vi "write_filter_spec.vi"(9 "IIR Filter Cluster":T1 {"Forward Coefficients" format="%#_4g"; "Reverse Coefficients" format="%#_4g"}, 11 "File path":path) -> (1 "Output matrix":dbl[][](array[numeric]) format="%0.3f")   [LabVIEW 2010]
uses:
  <vilib>/Utility/file.llb/Write To Spreadsheet File (DBL).vi
panel:
  # "Write out an IIR second order sections filter in the Matlab zpk2sos format.\n\nNote that in Labview terminology, with the transfer function b/a, b (the numerator) is  the \"Forward Coefficients\" and a (the denominator) is the \"Reverse Coefficients\"."
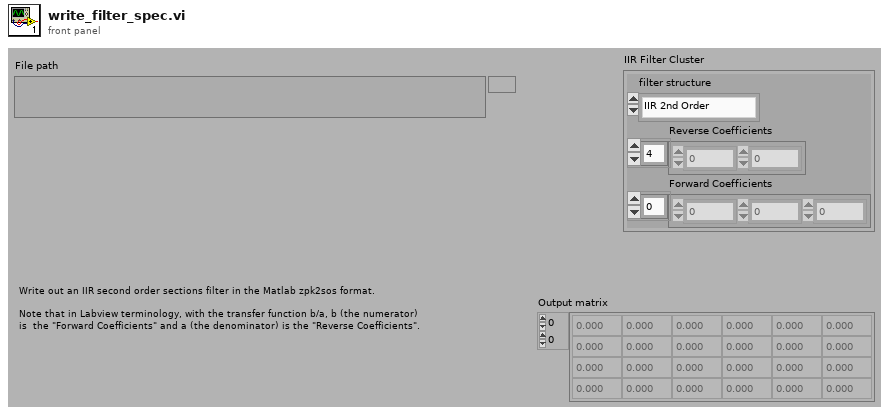
[diagram p1: front panel]
types:
  T1 = cluster{"filter structure":enum32{"IIR 2nd Order", "IIR 4th Order"}, "Reverse Coefficients":dbl[], "Forward Coefficients":dbl[]}
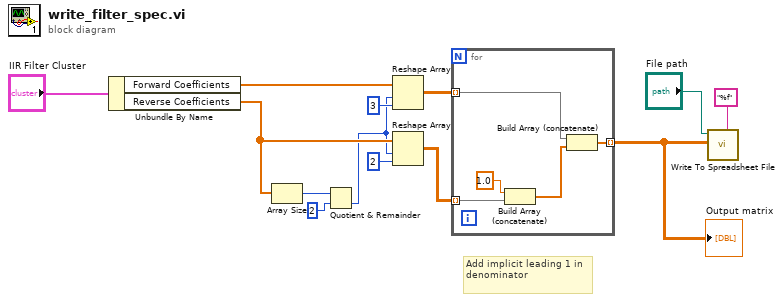
[diagram p0: block diagram]
diagram:
  # "Add implicit leading 1 in denominator"
  n1 = Unbundle By Name("IIR Filter Cluster") -> ("Forward Coefficients"=w8:dbl[], "Reverse Coefficients"=w9:dbl[])
  n2 = Array Size(array=w9) -> (size(s)=w13:i32)
  n3 = Quotient & Remainder(x=w13, y=2) -> (floor(x/y)=w5:i32)  [unwired: 1 out]
  n4 = Reshape Array(w8, w5, 3 ("dimension size")) -> (w6:dbl[][])
  n5 = Reshape Array(w9, w5, 2 ("dimension size")) -> (w7:dbl[][])
  n6 = for {
    tunnel: w7 -> [w18] mode=indexing
    tunnel: w6 -> [w14] mode=indexing
    tunnel: [w15] -> w2 mode=indexing
    n7 = Build Array (concatenate)(1.0 ("Fs"), w18) -> (w16:dbl[])
    n8 = Build Array (concatenate)(w14, w16) -> (w15:dbl[])
  }
  "Output matrix" <- w2
  n9 = call-poly <vilib>:"Write To Spreadsheet File.vi"("format (%.3f)"="%f", "2D data"=w2, "file path (dialog if empty)"="File path") -> ()  [unwired: 5 in, 1 out]
